vi "st_Geometric Inverse CDF (kx).vi"(10 "p":dbl=0.02, 11 "cdf(nx)":dbl=0.5) -> (0 "error":i32, 3 "nx":dbl=33.30961850946567)   [LabVIEW 2024, in "NI_Gmath.lvlib"]
uses:
  NI_Gmath.lvlib
  st_error_code.ctl
panel:
  # "Geometric Inverse CDF (kx)"
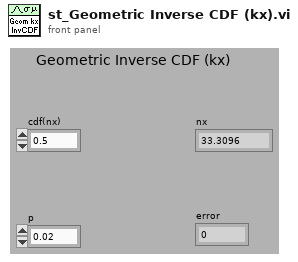
[diagram p1: front panel]
types:
  T1 = typedef "NI_Gmath.lvlib/st_error_code.ctl" = i32
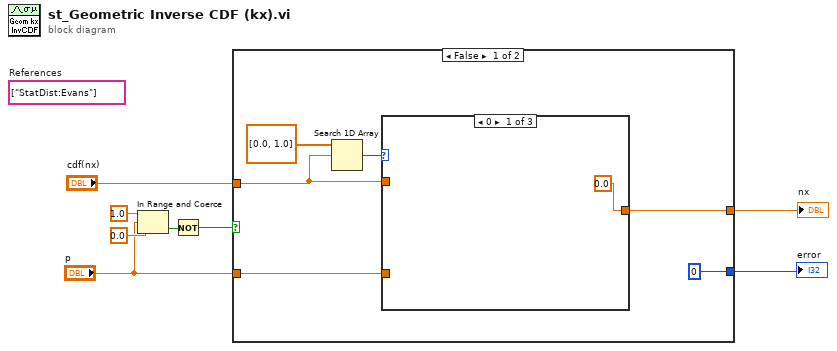
[diagram p0: block diagram]
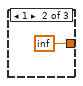
[diagram p2: hidden frame]
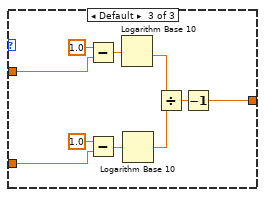
[diagram p3: hidden frame]
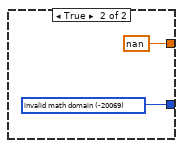
[diagram p4: hidden frame]
diagram:
  (unwired) string[] ["StatDist:Evans"]  # References
  n1 = In Range and Coerce(upper limit=1.0, x="p", lower limit=0.0) -> (In Range?=w3:bool)  [unwired: 1 out]
  n2 = Not(x=w3) -> (.not. x?=w1:bool)
  n3 = case shown="False" w1 {
    tunnel: "p" -> [w10 _]
    tunnel: [0 ("invalid math domain") w27] -> w8
    tunnel: [w9 nan] -> w7
    tunnel: "cdf(nx)" -> [w11 _]
    frame False {
      n4 = Search 1D Array(1D array=dbl[] [0.0, 1.0], element=w11) -> (index of element=w12:i32)  [unwired: 1 in]
      n5 = case shown="0" w12 {
        tunnel: [0.0 inf w18] -> w9
        tunnel: w11 -> [_ _ w17]
        tunnel: w10 -> [_ _ w23]
        frame 0 {
        }
        frame 1 {
        }
        frame Default {
          n6 = Subtract(x=1.0, y=w17) -> (x-y=w25:dbl)
          n7 = Subtract(x=1.0, y=w23) -> (x-y=w22:dbl)
          n8 = Logarithm Base 10(1:w25) -> (0:w21:dbl)
          n9 = Logarithm Base 10(1:w22) -> (0:w20:dbl)
          n10 = Divide(x=w21, y=w20) -> (x/y=w19:dbl)
          n11 = Decrement(x=w19) -> (x-1=w18:dbl)
        }
      }
    }
    frame True {
      w27 = T1 -20069 items=["invalid math domain"=-20069, "Fourier interpolation size m >= n"=-20070, "empty array"=-20003] ("stat interp error code")
    }
  }
  "nx" <- w7
  "error" <- w8
